vi "PPG_ABC.byte array 2 pattern data.vi"(1 "byteArray":T1, 5 "error in (no error)":errorcluster) -> (15 "byteArray out":T1, 17 "PGData out":T2, 19 "error out":errorcluster)   [LabVIEW 2014, in "PPG_ABC.lvlib"]
doc: "Converts data from a byte array to \"PGDataType\". This method is specific for using user defined patterns constructed of characters as used by the MM6 class."
uses:
  PPG_ABC.lvlib
  PPG_ABC.PG_dataType.ctl
  CSCore/CSSystem/CoreDefs/CoreDefs.rawDataType.ctl
  CSCore/CSSystem/CoreLib/CoreLib.byte array 2 string.vi
  CSCore/CSSystem/CoreLib/CoreLib.byte array 2 int.vi
  CSCore/CSSystem/CoreLib/CoreLib.byte array 2 double array.vi
  CSCore/CSSystem/CoreLib/CoreLib.lvlib
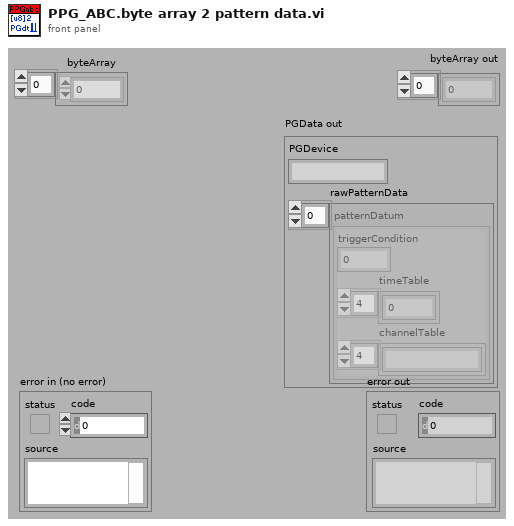
[diagram p1: front panel]
types:
  T1 = typedef "CoreDefs.rawDataType.ctl" = i8[]
  T2 = typedef "PPG_ABC.lvlib/PPG_ABC.PG_dataType.ctl" = cluster{"PGDevice":string, "rawPatternData":cluster{"triggerCondition":i32, "timeTable":dbl[], "channelTable":string[]}[]}
  T3 = cluster{"triggerCondition":i32, "timeTable":dbl[], "channelTable":string[]}[]
  T4 = cluster{"triggerCondition":i32, "timeTable":dbl[], "channelTable":string[]}
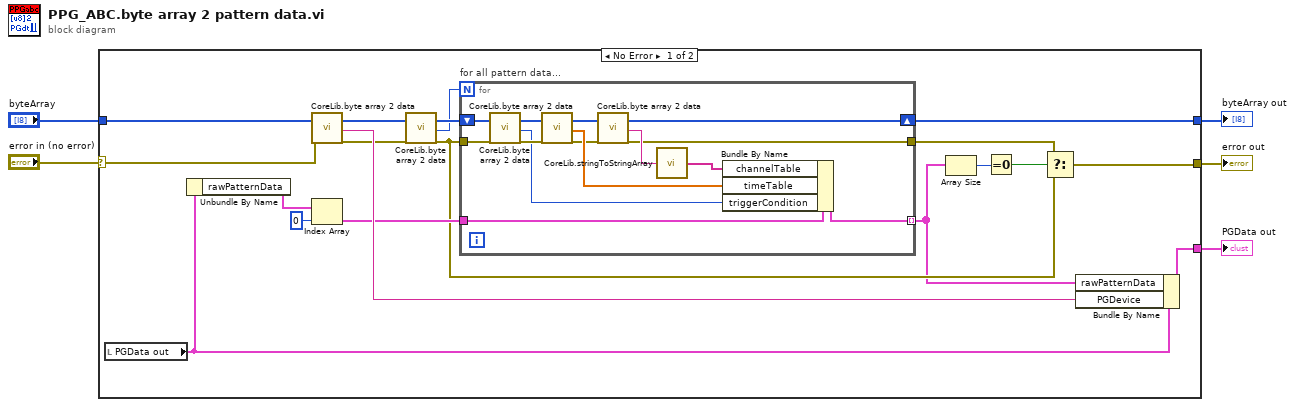
[diagram p0: block diagram]
diagram:
  n1 = case shown="No Error" "error in (no error)" {
    selector: "error in (no error)" -> [w14 w40]
    tunnel: "byteArray" -> [w24 w39]
    tunnel: [w18 _] -> w4
    tunnel: [w15 w40] -> w3
    tunnel: [w9 w39] -> w1
    frame No Error {
      n2 = local read "PGData out"() -> (w22:T2)
      n3 = Unbundle By Name(w22) -> ("rawPatternData"=w21:T3)
      n4 = call-poly "CoreLib.byte array 2 data.vi"("byteArray"=w24, "error in (no error)"=w14) -> ("byteArray out"=w10:T1, "string"=w23:string, "error out"=w13:errorcluster)  [unwired: 15 in]
      n5 = Index Array(array=w21, index=0) -> (element=w19:T4)
      n6 = call-poly "CoreLib.byte array 2 data.vi"("byteArray"=w10, "error in (no error)"=w13) -> ("byteArray out"=w11:T1, "i32"=w8:i32, "error out"=w12:errorcluster)  [unwired: 15 in]
      n7 = for "for all pattern data..." {
        N: w8 -> [_]
        shift-right: [w27] -> w9
        shift-left: w11 -> [w37]
        tunnel: w12 -> [w36]
        tunnel: [w25] -> w16
        tunnel: w19 -> [w38]
        tunnel: [w26] -> w7 mode=indexing
        n8 = call-poly "CoreLib.byte array 2 data.vi"("byteArray"=w37, "error in (no error)"=w36) -> ("byteArray out"=w34:T1, "i32"=w29:i32, "error out"=w35:errorcluster)  [unwired: 15 in]
        n9 = call-poly "CoreLib.byte array 2 data.vi"("byteArray"=w34, "error in (no error)"=w35) -> ("byteArray out"=w32:T1, "[d64]"=w33:dbl[], "error out"=w31:errorcluster)  [unwired: 15 in]
        n10 = call-poly "CoreLib.byte array 2 data.vi"("byteArray"=w32, "error in (no error)"=w31) -> ("byteArray out"=w27:T1, "string"=w30:string, "error out"=w25:errorcluster)  [unwired: 15 in]
        n11 = call "CoreLib.stringToStringArray.vi"("String"=w30) -> ("Array"=w28:string[])
        n12 = Bundle By Name(cluster=w38, "channelTable"=w28, "timeTable"=w33, "triggerCondition"=w29) -> (w26:T4)
      }
      n13 = Array Size(array=w7) -> (size(s)=w6:i32)
      n14 = Equal To 0?(x=w6) -> (x = 0?=w17:bool)
      n15 = Select(t=w16, s=w17, f=w12) -> (s? t:f=w15:errorcluster)
      n16 = Bundle By Name(cluster=w22, "rawPatternData"=w7, "PGDevice"=w23) -> (w18:T2)
    }
    frame Error {
    }
  }
  "PGData out" <- w4
  "error out" <- w3
  "byteArray out" <- w1
